vi "PH_SSAC.calc Pulse Duration.vi"(0 "Peak Duration [pixel]":dbl, 1 "Calibration Factor [fs/pixel]":dbl) -> (2 "Pulse Duration [fs]":dbl)   [LabVIEW 2014, in "PH_SSAC.lvlib"]
doc: "This VI calculates the pulse duration in femto seconds as follows:\n\nAbs value (Peak Duration [pixel] * Calibration Factor [fs/pixel] / sqrt(2))"
uses:
  PH_SSAC.lvlib
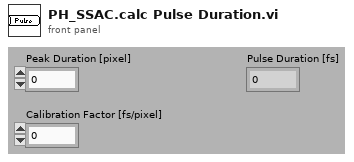
[diagram p1: front panel]
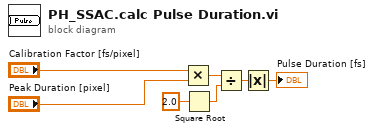
[diagram p0: block diagram]
diagram:
  n1 = Multiply(x="Calibration Factor [fs/pixel]", y="Peak Duration [pixel]") -> (x*y=w1:dbl)
  n2 = Square Root(x=2.0) -> (sqrt(x)=w3:dbl)
  n3 = Divide(x=w1, y=w3) -> (x/y=w4:dbl)
  n4 = Absolute Value(x=w4) -> (abs(x)=→"Pulse Duration [fs]":dbl)
